vi "GET-SET_POWER_LEVEL_1.0.0.vi"(1 "Max Power":dbl=-8.0, 4 "Delay After Set (ms)":dbl=1.0 format="%#_13g", 5 "Offset(dB)":dbl, 6 "Get Power Only (T)":bool, 7 "Skip(T)":bool, 8 "error in":errorcluster {"code" format="%.0x"}, 9 "Timeout":u32=3000, 10 "Power(dB)":dbl, 11 "Session In":refnum<visa-resource-name>="GPIB0::22::INSTR") -> (0 "error out":errorcluster {"code" format="%.0x"}, 2 "Get Power":dbl, 3 "Session Out":refnum<visa-resource-name>)   [LabVIEW 2018]
uses:
  <vilib>/Utility/error.llb/DialogType.ctl
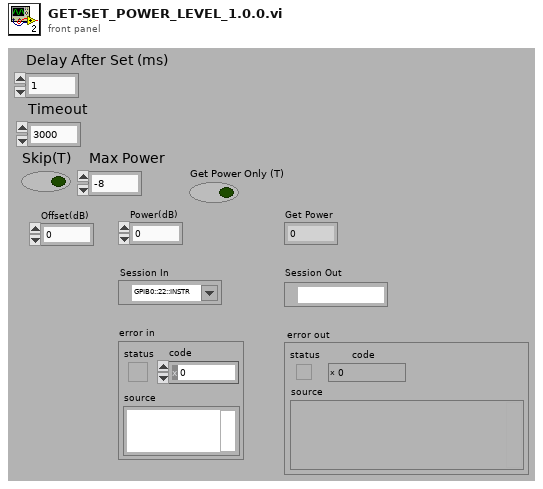
[diagram p1: front panel]
types:
  T1 = typedef "DialogType.ctl" = u16
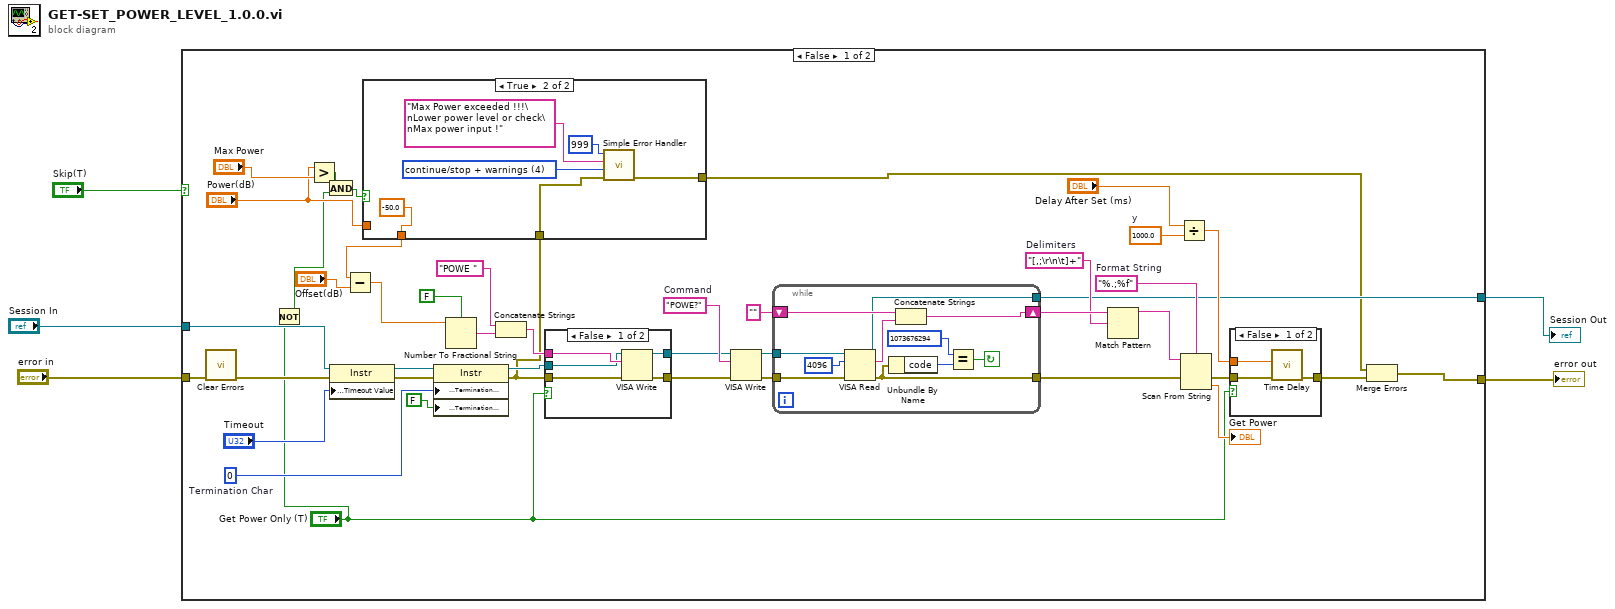
[diagram p0: block diagram]
diagram:
  n1 = case shown="False" "Skip(T)" {
    tunnel: "error in" -> [w48 w79]
    tunnel: "Session In" -> [w45 w80]
    tunnel: [w11 w79] -> w3
    tunnel: [w19 w80] -> w2
    frame False {
      w21 = 1000.0  # y
      w27 = "[,;\r\n\t]+"  # Delimiters
      w29 = "%.;%f"  # Format String
      w32 = "POWE?"  # Command
      w43 = u8 0  # Termination Char
      n2 = call <vilib>:"Clear Errors.vi"("error in (no error)"=w48) -> ("error out"=w13:errorcluster)  [unwired: 5 in, 1 out]
      n3 = Not(x="Get Power Only (T)") -> (.not. x?=w6:bool)
      n4 = Greater?(x="Power(dB)", y="Max Power") -> (0:w9:bool)
      n5 = And(x=w9, y=w6) -> (x .and. y?=w8:bool)
      n6 = property class="Instr"(reference=w45, error in=w13, "General Settings:Timeout Value"="Timeout") -> (reference out=w42:refnum<visa-resource-name>, error out=w44:errorcluster)
      n7 = property class="Instr"(reference=w42, error in=w44, "Message Based Settings:Termination Character"=w43, "Message Based Settings:Termination Character Enable"=FALSE ("enable")) -> (reference out=w26:refnum<visa-resource-name>, error out=w12:errorcluster)
      n8 = case shown="True" w8 {
        tunnel: [w49 w56] -> w10
        tunnel: [w50 -50.0] -> w15
        tunnel: "Power(dB)" -> [w50 _]
        tunnel: w12 -> [w49 w51]
        frame False {
        }
        frame True {
          w53 = T1 4 items=["no dialog", "OK message", "continue or stop message", "OK message + warnings", "continue/stop + warnings"] ("type of dialog (OK msg:1)")
          n9 = call <vilib>:"Simple Error Handler.vi"("error code (no error:0)"=999, "error source (\" \")"="Max Power exceeded !!!\nLower power level or check\nMax power input !" ("error source (\" \")"), "type of dialog (OK msg:1)"=w53, "error in (no error)"=w51) -> ("error out"=w56:errorcluster)  [unwired: 1 in, 4 out]
        }
      }
      n10 = Subtract(x=w15, y="Offset(dB)") -> (x-y=w17:dbl)
      n11 = Number To Fractional String(use system decimal point (T)=FALSE, number=w17) -> (F-format string=w40:string)  [unwired: 2 in]
      n12 = Concatenate Strings("POWE " ("staticText"), w40) -> (w37:string)
      n13 = case shown="False" "Get Power Only (T)" {
        tunnel: w12 -> [w65 w67]
        tunnel: [w64 w67] -> w38
        tunnel: w37 -> [w63 _]
        tunnel: w26 -> [w62 w66]
        tunnel: [w61 w66] -> w20
        frame False {
          n14 = VISA Write(VISA resource name=w62, write buffer=w63, error in (no error)=w65) -> (VISA resource name out=w61:refnum<visa-resource-name>, error out=w64:errorcluster)  [unwired: 1 out]
        }
        frame True {
        }
      }
      n15 = VISA Write(VISA resource name=w20, write buffer=w32, error in (no error)=w38) -> (VISA resource name out=w36:refnum<visa-resource-name>, error out=w35:errorcluster)  [unwired: 1 out]
      n16 = while {
        tunnel: w36 -> [w75]
        shift-right: [w69] -> w31
        shift-left: "" -> [w74]
        tunnel: w35 -> [w72]
        tunnel: [w71] -> w34
        tunnel: [w68] -> w19
        stop <- w70 continue-if-true
        n17 = VISA Read(VISA resource name=w75, byte count=u32 4096 ("byte count (0)"), error in (no error)=w72) -> (VISA resource name out=w68:refnum<visa-resource-name>, read buffer=w73:string, error out=w71:errorcluster)  [unwired: 1 out]
        n18 = Unbundle By Name(w71) -> ("code"=w77:i32)
        n19 = Concatenate Strings(w74, w73) -> (w69:string)
        n20 = Equal?(x=1073676294, y=w77) -> (x = y?=w70:bool)
      }
      n21 = Match Pattern(string=w31, regular expression=w27) -> (before substring=w30:string)  [unwired: 1 in, 3 out]
      n22 = Divide(x="Delay After Set (ms)", y=w21) -> (x/y=w22:dbl)
      n23 = Scan From String(format string=w29, input string=w30, error in=w34) -> (error out=w24:errorcluster, output 1=→"Get Power":dbl)  [unwired: 2 in, 2 out]
      n24 = case shown="False" "Get Power Only (T)" {
        tunnel: [w59 w60] -> w25
        tunnel: w24 -> [w58 w60]
        tunnel: w22 -> [w57 _]
        frame False {
          n25 = call "Time Delay"("error in (no error)"=w58, "Delay Time (s)"=w57) -> ("error out"=w59:errorcluster)  [unwired: 9 in]
        }
        frame True {
        }
      }
      n26 = Merge Errors(w10, w25) -> (w11:errorcluster)
    }
    frame True {
    }
  }
  "error out" <- w3
  "Session Out" <- w2
